vi "Periodic Tasks.vi"(8 "error in":errorcluster) -> ()   [LabVIEW 2016]
doc: "This VI runs in parallel to other tasks. It can contain as many user-defined periodic loops as you need. These can carry out PID or other sorts of timed response."
uses:
  Systems/Joystick/Joystick.lvlib
  Systems/WC_Drive/WC_Drive.lvlib
  Systems/Compressor/Compressor.lvlib
  Systems/Dashboard/DashboardComm.lvlib
  Systems/System_Monitoring/System_Status.lvlib
  Systems/Gear Pickup/Gear Pickup.lvlib
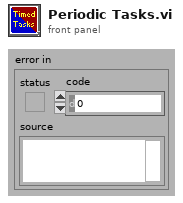
[diagram p1: front panel]
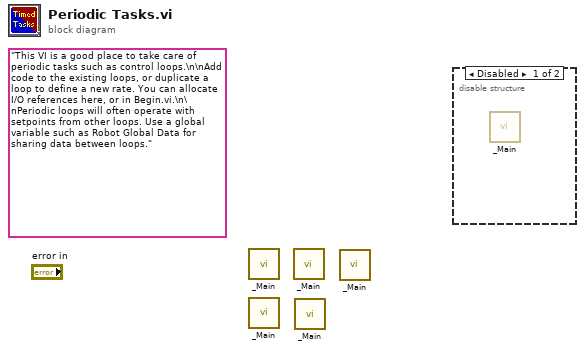
[diagram p0: block diagram]
diagram:
  (unwired) "This VI is a good place to take care of periodic tasks such as control loops.\n\nAdd code to the existing loops, or duplicate a loop to define a new rate. You can allocate I/O references here, or in Begin.vi.\n\nPeriodic loops will often operate with setpoints from other loops. Use a global variable such as Robot Global Data for sharing data between loops."
  n1 = call "_Main.vi"() -> ()  [unwired: 12 in]
  n2 = call "_Main.vi"() -> ()  [unwired: 12 in]
  n3 = call "_Main.vi"() -> ()  [unwired: 12 in]
  n4 = call "_Main.vi"() -> ()  [unwired: 12 in]
  n5 = call "_Main.vi"() -> ()  [unwired: 12 in]
  n6 = disable-structure shown="Disabled" {
    frame Disabled {
      n7 = call "_Main.vi"() -> ()  [unwired: 12 in]
    }
    frame Enabled {
    }
  }
